vi "Set Trace Step.vi"(7 "Processing Step":T1=enum."Request", 11 "Processing in":refnum<class "Processing.lvclass">) -> (3 "Processing out":refnum<class "Processing.lvclass">)   [LabVIEW 2020, in "HTTP Server.lvlib" / "Processing.lvclass"]
uses:
  Processing.lvclass
  Processing Step.ctl
  Processing.lvclass/Processing.ctl
  RequestTraceLog/RequestTraceLog.lvclass
  HTTP Server.lvlib
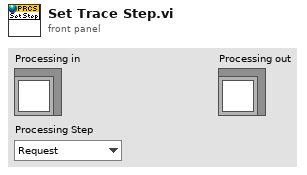
[diagram p1: front panel]
types:
  T1 = typedef "HTTP Server.lvlib/Processing Step.ctl" = enum16{"Connection", "Request", "Routing", "Controller Init", "Controller", "Response", "Complete", "Exception"}
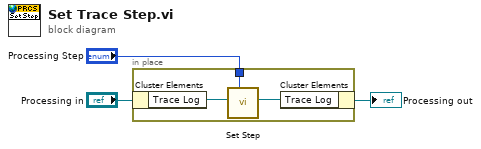
[diagram p0: block diagram]
diagram:
  n1 = in-place {
    in-place-border: "Processing Step" -> [w6]
    n2 = in-place-cluster #1("Processing in") -> ("Trace Log"=w5:refnum<class "RequestTraceLog.lvclass">)
    n3 = call "Set Step.vi"("Processing Step"=w6, "RequestTraceLog in"=w5) -> ("RequestTraceLog out"=w4:refnum<class "RequestTraceLog.lvclass">)  [unwired: 9 in]
    n4 = in-place-cluster #1("Trace Log"=w4) -> (→"Processing out":refnum<class "Processing.lvclass">)
  }
